vi "Put-Ball-Pro_Test.vi"() -> ()   [LabVIEW 2019]
uses:
  <vilib>/myRIO/Common/Instrument Driver Framework/myRIO v1.0/UART/vis/myRIO v1.0 Close UART.vi
  Variable/Go-Home.vi
  <vilib>/myRIO/Common/Instrument Driver Framework/Utilities/vis/FPGA Ref Manager.vi
  <vilib>/myRIO/Common/Instrument Driver Framework/myRIO v1.0/myRIO v1.0 Reset FPGA.vi
  <vilib>/myRIO/Common/Instrument Driver Framework/myRIO v1.0/IRQ/vis/myRIO v1.0 IRQ Info FGV.vi
  <vilib>/myRIO/Common/Instrument Driver Framework/myRIO v1.0/IRQ/vis/myRIO v1.0 Timer IRQ Info FGV.vi
  <vilib>/myRIO/Common/Instrument Driver Framework/myRIO v1.0/IRQ/vis/myRIO v1.0 ISR Agent.vi
  <vilib>/myRIO/Instrument Drivers/Utilities/vis/Reset Index.vi
  <vilib>/myRIO/Common/Instrument Driver Framework/myRIO v1.0/Resource Manager/vis/myRIO v1.0 Block Write Resource Manager.vi
  <vilib>/myRIO/Instrument Drivers/Utilities/Utilities.lvlib
panel:
  in  "Error In":errorcluster
  out "當前動作":enum16{"一二", "一三", "一四", "二三", "二四", "三四"}(ring)
  in  "Stop":bool
  out "Error Out":errorcluster
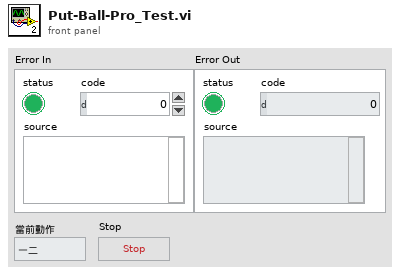
[diagram p1: front panel]
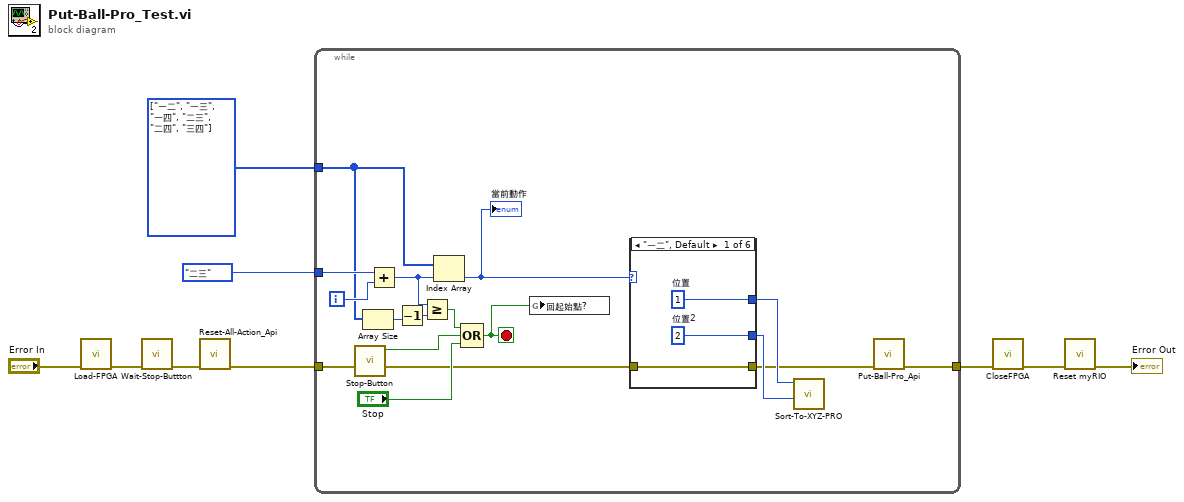
[diagram p0: block diagram]
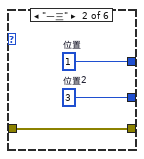
[diagram p2: hidden frame]
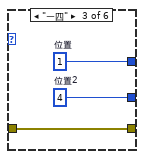
[diagram p3: hidden frame]
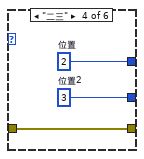
[diagram p4: hidden frame]
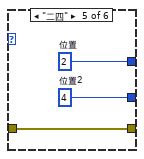
[diagram p5: hidden frame]
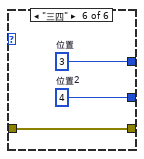
[diagram p6: hidden frame]
diagram:
  w3 = enum16{"一二", "一三", "一四", "二三", "二四", "三四"}[] [enum."一二", enum."一三", enum."一四", enum."二三", enum."二四", enum."三四"] items=["一二", "一三", "一四", "二三", "二四", "三四"]
  n1 = call "Load-FPGA.vi"("Error In"="Error In") -> ("Error Out"=w6:errorcluster)  [unwired: 10 in]
  n2 = call "Wait-Stop-Buttton.vi"("Error In"=w6) -> ("Error Out"=w5:errorcluster)  [unwired: 10 in]
  n3 = call "Reset-All-Action_Api.vi"("Error In"=w5) -> ("Error Out"=w4:errorcluster)  [unwired: 8 in, 2 out]
  n4 = while {
    tunnel: w4 -> [w12]
    tunnel: enum16{"一二", "一三", "一四", "二三", "二四", "三四"}."二三" -> [w24]
    tunnel: w3 -> [w18]
    tunnel: [w11] -> w1
    i -> [w25]
    stop <- w15 stop-if-true
    n5 = call "Stop-Button.vi"() -> ("顯示按下?"=w19:bool)  [unwired: 10 in, 1 out]
    n6 = Array Size(array=w18) -> (size(s)=w21:i32)
    n7 = Add(x=w24, y=w25) -> (x+y=w16:i32)
    n8 = Decrement(x=w21) -> (x-1=w20:i32)
    n9 = Greater Or Equal?(x=w16, y=w20) -> (x >= y?=w22:bool)
    n10 = Index Array(array=w18, index=w16) -> (element=w23:enum16{"一二", "一三", "一四", "二三", "二四", "三四"})
    "當前動作" <- w23
    n11 = Compound Arithmetic op=OR(w22, w19, "Stop") -> (w15:bool)
    n12 = global write "Go-Home.vi" "回起始點?"(w15) -> ()
    n13 = case shown="\"一二\", Default" w23 {
      tunnel: [w28 w31 w34 w37 w40 w43] -> w14
      tunnel: [w27 w30 w33 w36 w39 w42] -> w13
      tunnel: [w26 w29 w32 w35 w38 w41] -> w10
      tunnel: w12 -> [w26 w29 w32 w35 w38 w41]
      frame "一二", Default {
        w27 = 2  # 位置2
        w28 = 1  # 位置
      }
      frame "一三" {
        w30 = 3  # 位置2
        w31 = 1  # 位置
      }
      frame "一四" {
        w33 = 4  # 位置2
        w34 = 1  # 位置
      }
      frame "二三" {
        w36 = 3  # 位置2
        w37 = 2  # 位置
      }
      frame "二四" {
        w39 = 4  # 位置2
        w40 = 2  # 位置
      }
      frame "三四" {
        w42 = 4  # 位置2
        w43 = 3  # 位置
      }
    }
    n14 = call "Sort-To-XYZ-PRO.vi"("位置 2"=w13, "位置"=w14) -> ()  [unwired: 7 in, 3 out]
    n15 = call "Put-Ball-Pro_Api.vi"("Error In"=w10) -> ("Error Out"=w11:errorcluster)  [unwired: 9 in, 1 out]
  }
  n16 = call "CloseFPGA.vi"("Error In"=w1) -> ("Error Out"=w9:errorcluster)  [unwired: 10 in]
  n17 = call <vilib>:"Reset myRIO.vi"("error in (no error)"=w9) -> ("error out"=→"Error Out":errorcluster)  [unwired: 10 in]
